vi "setComment.vi"(8 "error in (no error)":errorcluster, 10 "comment":string, 11 "RampEvent.lvclass in":refnum<class "RampEvent.lvclass">) -> (0 "error out":errorcluster, 3 "RampEvent.lvclass out":refnum<class "RampEvent.lvclass">)   [LabVIEW 2009, in "Tools.lvlib" / "Scripting.lvlib" / "RampEvent.lvclass"]
uses:
  RampEvent.lvclass
  ScriptEvent.lvclass
  RampEvent.lvclass/RampEvent.ctl
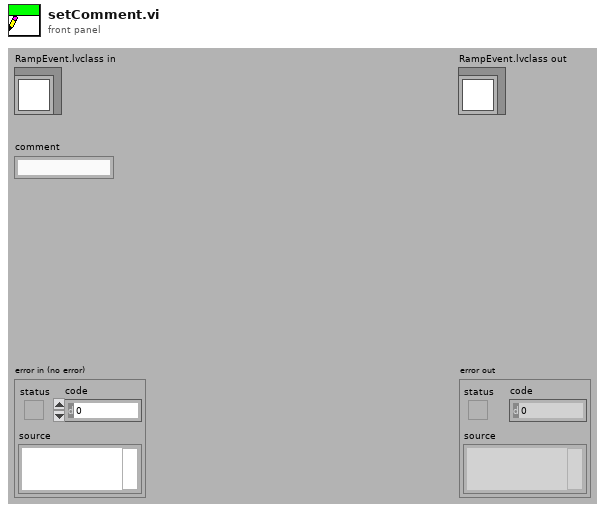
[diagram p1: front panel]
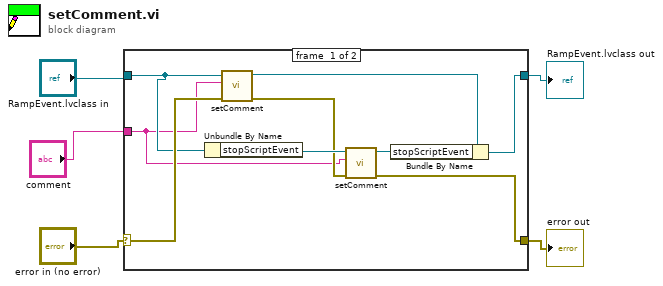
[diagram p0: block diagram]
diagram:
  n1 = case shown="No Error" "error in (no error)" {
    selector: "error in (no error)" -> [w14 w15]
    tunnel: [w6 w15] -> w1
    tunnel: "RampEvent.lvclass in" -> [w13 w16]
    tunnel: [w7 w16] -> w4
    tunnel: "comment" -> [w10 _]
    frame #0 {
      n2 = Unbundle By Name(w13) -> ("stopScriptEvent"=w12:refnum<class "ScriptEvent.lvclass">)
      n3 = call-parent "setComment.vi"("error in (no error)"=w14, "comment"=w10, "ScriptEvent.lvclass in"=w13) -> ("error out"=w11:errorcluster, "ScriptEvent.lvclass out"=w9:refnum<class "RampEvent.lvclass">)  [unwired: 7 in]
      n4 = call-parent "setComment.vi"("error in (no error)"=w11, "comment"=w10, "ScriptEvent.lvclass in"=w12) -> ("error out"=w6:errorcluster, "ScriptEvent.lvclass out"=w8:refnum<class "ScriptEvent.lvclass">)  [unwired: 7 in]
      n5 = Bundle By Name(cluster=w9, "stopScriptEvent"=w8) -> (w7:refnum<class "RampEvent.lvclass">)
    }
    frame #1 {
    }
  }
  "error out" <- w1
  "RampEvent.lvclass out" <- w4
